vi "pm Main.vi"() -> ()   [LabVIEW 2022 SP3]
doc: "This Continuous Measurement sample project is based on the Queued Message Handler template.\n\nThe Event Handling Loop generates messages based on user interface actions.\n\nThe Message Handling Loop processes messages generated by the Event Handling Loop, or by other messages. There are also Acquisition and Logging message handling loop subVIs, and a chart updating loop."
uses:
  Settings/Settings.ctl
  Acquisition/Hardware Configuration.ctl
  Acquisition/Signal Type.ctl
  Logging/Logging Configuration.ctl
  controls/pm UI Data.ctl
  controls/pm UI State.ctl
  support/Message Queue/Enqueue Message (Single).vi
  support/Message Queue/Enqueue Message (Array).vi
  <vilib>/Utility/error.llb/Error Cluster From Error Code.vi
  <vilib>/ErrorRing/Error Ring.xnode
  Acquisition/pm Acquisition.lvlib
  Logging/pm Logging.lvlib
  Settings/pm Settings.lvlib
  support/User Event - Stop/pm User Event - Stop.lvlib
  support/Message Queue/pm Message Queue.lvlib
  Settings/Settings Dialog.vi
panel:
  out "Message Data":variant
  out "averagedPower":string
  out "instantPower":string
  in  "wavelength":string="976" caption="wavelenght"
  in  "Save":bool
  in  "Start":bool
  in  "Stop":bool
  in  "Settings":bool
  in  "Exit":bool
  out "Status":string
  out "DIstributionP":dbl[][](graph) caption="Intensity Graph"
  out "Data":waveform(dbl)[](graph)
  # "Longueur d'onde"
  # "Yes\nNo\nToaster"
  # "nm"
  # "logo..."
  # "Puissance instantannée"
  # "W"
  # "Puissance moyenne"
  # "W"
  # "Distribution de puissance"
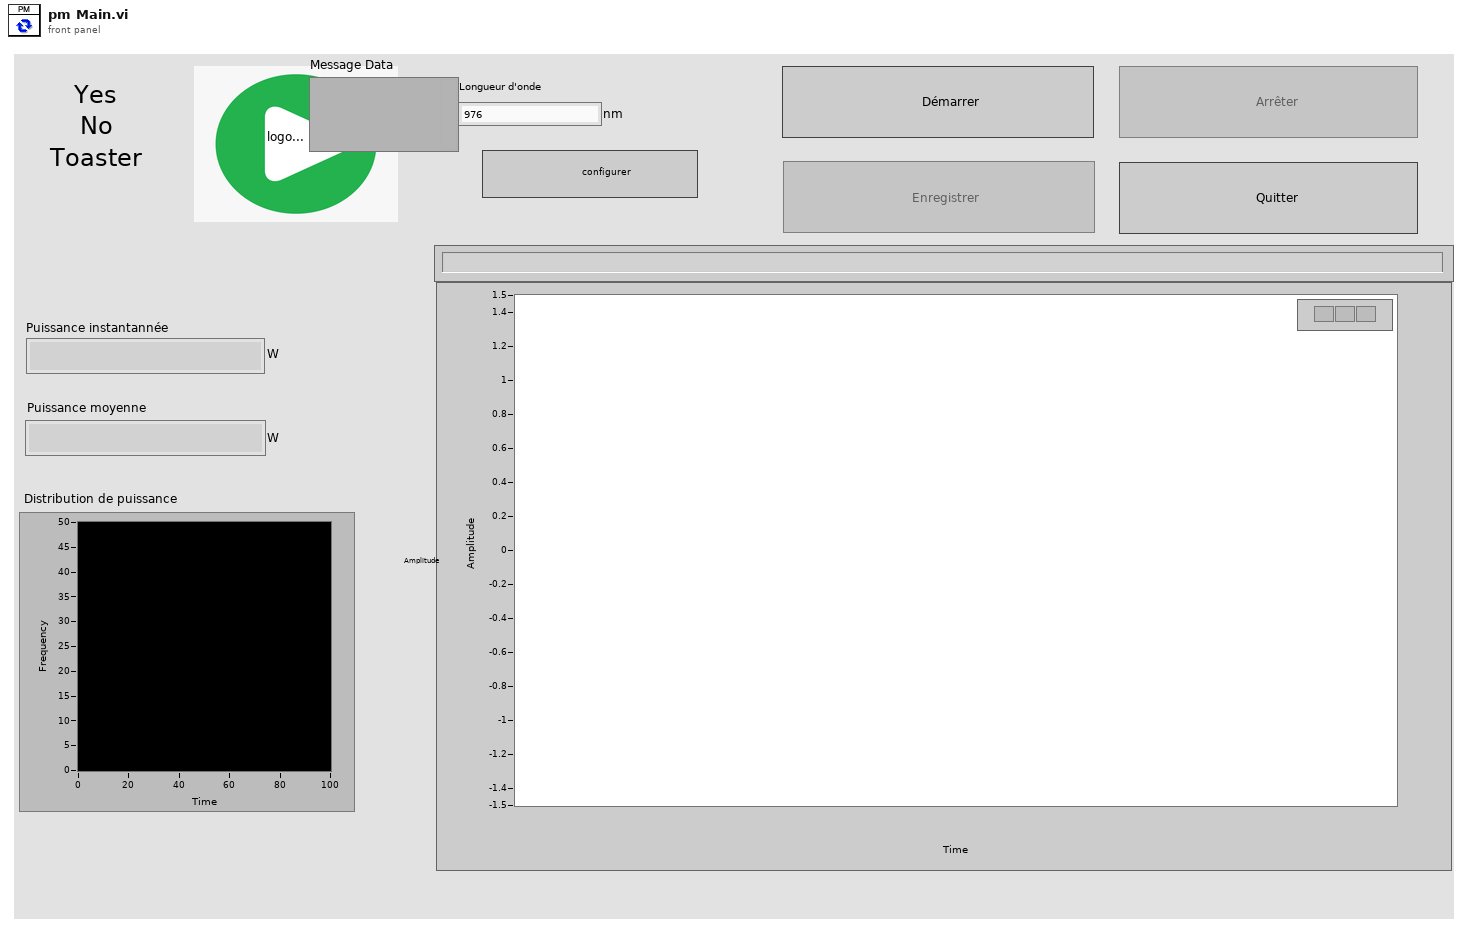
[diagram p1: front panel]
types:
  T1 = typedef "pm UI State.ctl" = enum16{"Idle", "Acquiring and Logging", "Waiting for Exit", "Waiting for Exit (Acq Stopped)", "Waiting for Exit (Log Stopped)", "Waiting for Stop", "Waiting for Stop (Acq Stopped)", "Waiting for Stop (Log Stopped)", "Saving data"}
  T2 = typedef "pm UI Data.ctl" = cluster{"Start Ref":refnum<vi>, "Stop Ref":refnum<vi>, "Settings Ref":refnum<vi>, "Exit Ref":refnum<vi>, "Status Ref":refnum<vi>, "Data Ref":refnum<vi>, "Save":refnum<vi>, "wavelength":refnum<vi>}
  T3 = typedef "pm Settings.lvlib/Settings.ctl" = cluster{"Hardware Configuration":T4, "Logging Configuration":T6}
  T4 = typedef "pm Acquisition.lvlib/Hardware Configuration.ctl" = cluster{"HW Refnum <Replace Me>":string, "Signal Type <Replace Me>":T5}
  T5 = typedef "pm Acquisition.lvlib/Signal Type.ctl" = enum16{"Sine Wave", "Square with Noise"}
  T6 = typedef "pm Logging.lvlib/Logging Configuration.ctl" = cluster{"Log File Base Path":path, "TDMS File Reference":refnum<k34>}
  T7 = typedef "pm Message Queue.lvlib/All Message Queues.ctl" = cluster{"UI":refnum<queue>, "Acquisition":refnum<queue>, "Logging":refnum<queue>}
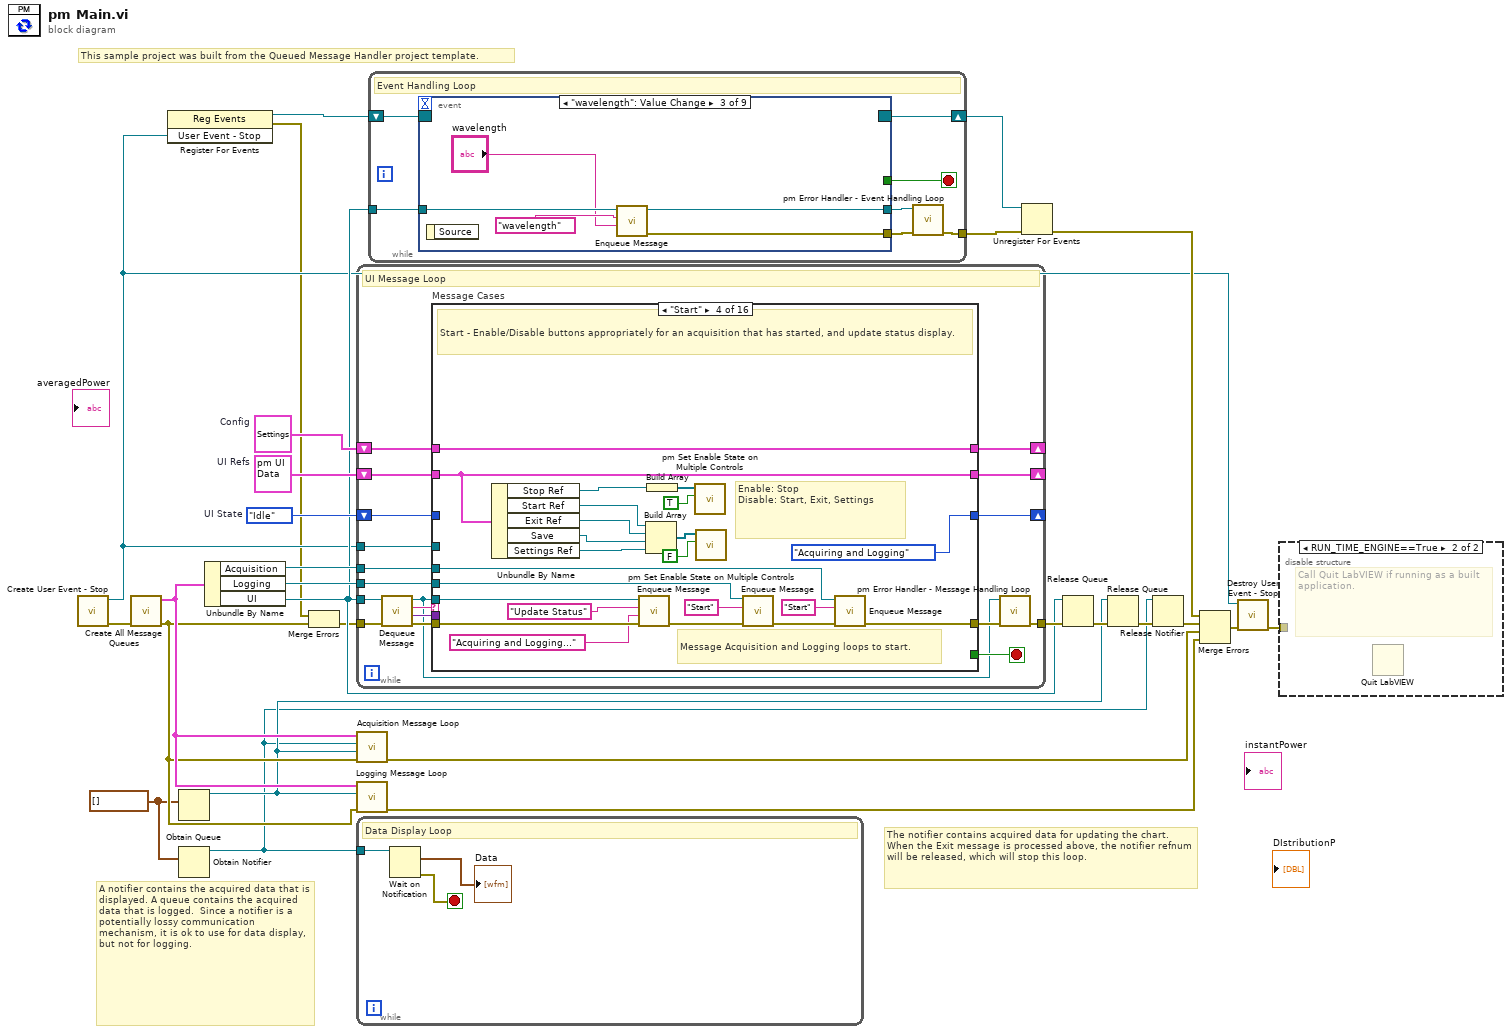
[diagram p0: block diagram]
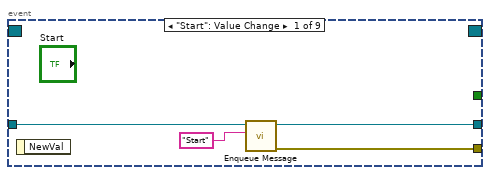
[diagram p3: hidden frame]
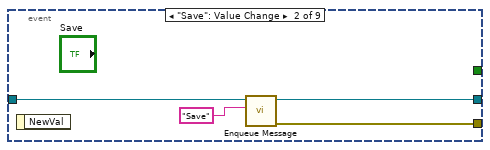
[diagram p4: hidden frame]
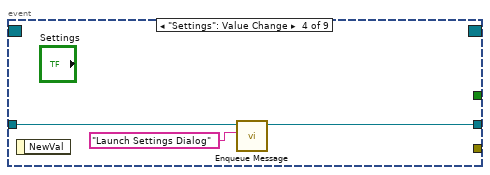
[diagram p5: hidden frame]
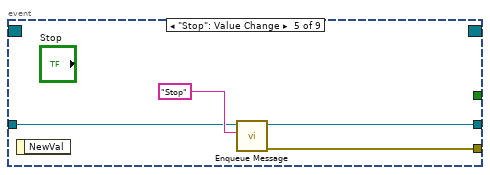
[diagram p6: hidden frame]
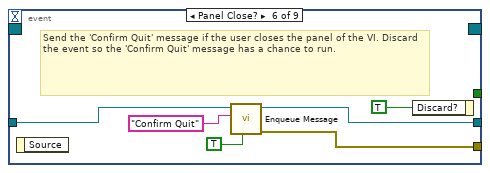
[diagram p7: hidden frame]
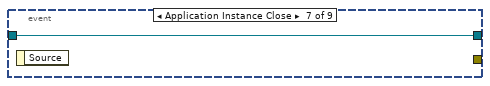
[diagram p8: hidden frame]
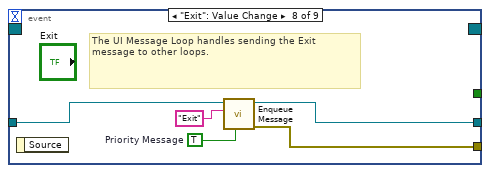
[diagram p9: hidden frame]
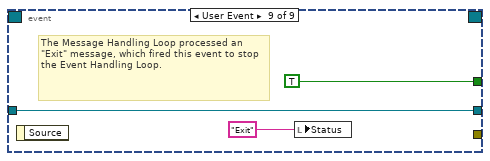
[diagram p10: hidden frame]
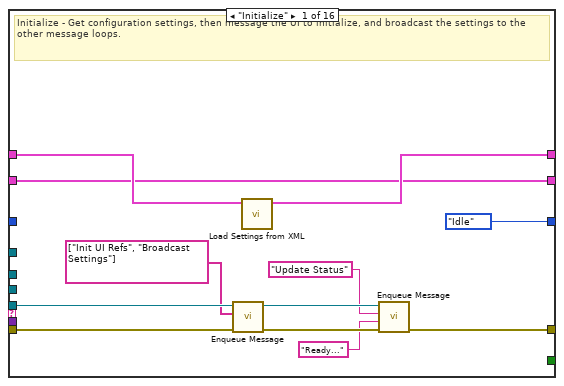
[diagram p11: hidden frame]
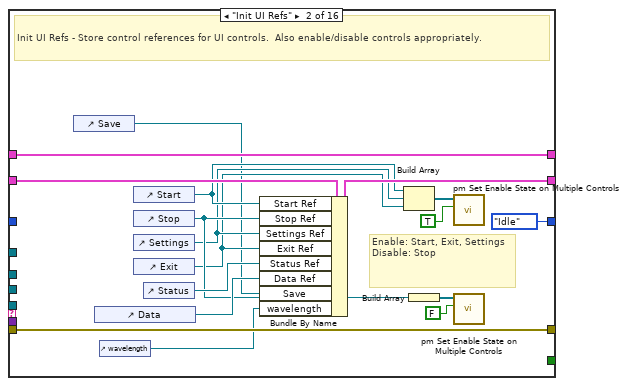
[diagram p12: hidden frame]
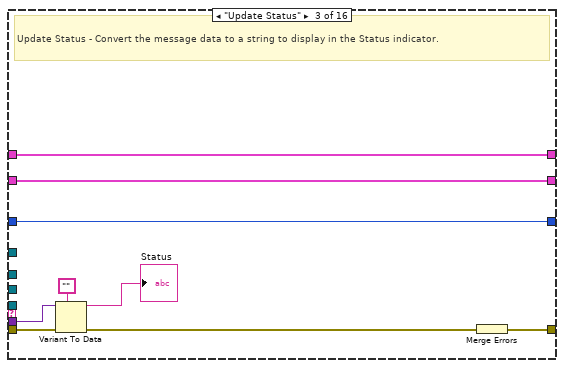
[diagram p13: hidden frame]
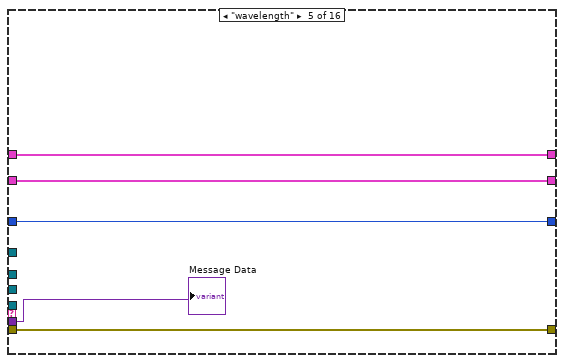
[diagram p14: hidden frame]
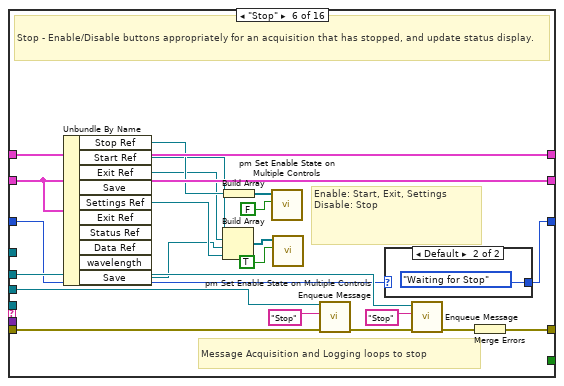
[diagram p15: hidden frame]
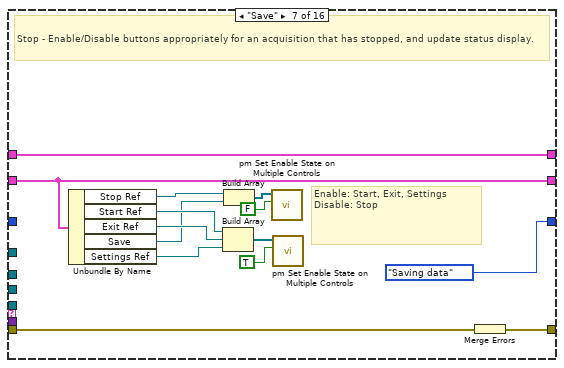
[diagram p17: hidden frame]
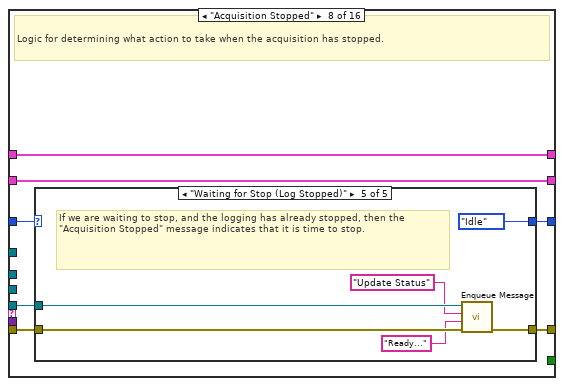
[diagram p18: hidden frame]
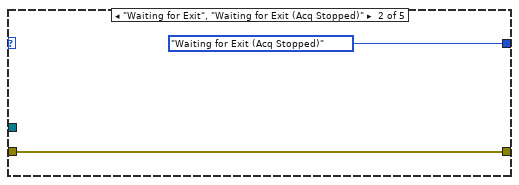
[diagram p20: hidden frame]
diagram:
  w14 = pm_UI_State."Idle"  # UI State
  w5 = waveform(dbl)[] []
  w17 = T2 {"Start Ref"=refnum, "Stop Ref"=refnum, "Settings Ref"=refnum, "Exit Ref"=refnum, "Status Ref"=refnum, "Data Ref"=refnum, "Save"=refnum, "wavelength"=refnum}  # UI Refs
  w20 = T3 {"Hardware Configuration"={"HW Refnum <Replace Me>"="", "Signal Type <Replace Me>"=enum."Sine Wave"}, "Logging Configuration"={"Log File Base Path"=path "", "TDMS File Reference"=refnum}}  # Config
  # "This sample project was built from the Queued Message Handler project template."
  # "A notifier contains the acquired data that is displayed. A queue contains the acquired data that is logged.  Since a notifier is a potentially lossy communication mechanism, it is ok to use for data display, but not for logging."
  # "The notifier contains acquired data for updating the chart. When the Exit message is processed above, the notifier refnum will be released, which will stop this loop."
  n1 = call "Create User Event - Stop.vi"() -> ("error out"=w24:errorcluster, "User Event - Stop"=w3:refnum<user-event>)  [unwired: 10 in]
  n2 = call "Create All Message Queues.vi"("error in (no error)"=w24) -> ("error out"=w21:errorcluster, "Message Queues out"=w23:T7)  [unwired: 9 in]
  n3 = register-events(w3) -> (reference out=w4:refnum<event-registration>, error out=w1:errorcluster)  [unwired: 2 in]
  n4 = Obtain Queue(element data type=w5) -> (queue out=w7:refnum<queue>)  [unwired: 4 in, 2 out]
  n5 = Obtain Notifier(notification data type=w5) -> (notifier out=w6:refnum<notifier>)  [unwired: 3 in, 2 out]
  n6 = Unbundle By Name(w23) -> ("Acquisition"=w16:refnum<queue>, "Logging"=w15:refnum<queue>, "UI"=w12:refnum<queue>)
  n7 = Merge Errors(w1, w21) -> (w2:errorcluster)
  n8 = while {
    tunnel: w12 -> [w39]
    tunnel: w3 -> [w44]
    shift-right: [w38] -> _
    shift-left: w20 -> [w37]
    shift-right: [w35] -> _
    shift-left: w17 -> [w36]
    tunnel: w16 -> [w34]
    tunnel: w15 -> [w33]
    shift-right: [w28] -> _
    shift-left: w14 -> [w29]
    tunnel: w2 -> [w43]
    tunnel: [w32] -> w27
    stop <- w45 stop-if-true
    # "UI Message Loop"
    n9 = call "Dequeue Message.vi"("error in (no error)"=w43, "Message Queue"=w39) -> ("error out"=w42:errorcluster, "Message Data"=w40:variant, "Message"=w41:string, "dup Message Queue"=w30:refnum<queue>)  [unwired: 6 in]
    n10 = case "Message Cases" shown="\"Start\"" w41 {
      selector: w41 -> [_ _ _ _ _ _ _ _ _ _ _ _ _ _ _ w284]
      tunnel: w30 -> [w49 _ _ w106 _ _ _ w151 w176 _ w216 _ w237 _ _ _]
      tunnel: w42 -> [w48 w74 w82 w105 w111 w131 w135 w152 w177 w204 w218 w225 w236 w265 w282 _]
      tunnel: [w53 w74 w83 w88 w111 w132 w148 w149 w174 w210 w211 w228 w235 w275 w281 w283] -> w31
      tunnel: [_ _ _ _ _ _ _ _ _ _ _ _ _ TRUE _ _] -> w45
      tunnel: w40 -> [_ _ w81 _ w107 _ _ _ _ _ _ w229 _ w263 _ _]
      tunnel: w44 -> [_ _ _ _ _ _ _ _ _ _ _ _ _ w276 _ _]
      tunnel: [w56 w73 w77 w104 w110 w130 w147 w155 w180 w208 w215 w233 w240 w274 w280 w287] -> w38
      tunnel: w37 -> [w57 w73 w77 w104 w110 w130 w147 w155 w180 w208 w219 w233 w240 w274 w280 w287]
      tunnel: w36 -> [w50 w72 w76 w101 w108 w129 w146 w154 w179 w202 w213 w232 w239 w273 w279 w286]
      tunnel: [w50 w69 w76 w101 w108 w129 w146 w154 w179 w202 w213 w232 w239 w273 w279 w286] -> w35
      tunnel: w34 -> [_ _ _ w87 _ w116 _ _ _ w201 _ _ _ w272 _ _]
      tunnel: w33 -> [_ _ _ w90 _ w119 _ _ _ w200 _ _ _ w271 _ _]
      tunnel: w29 -> [_ _ w75 _ w109 w113 _ w153 w178 w199 w212 w227 w238 _ w278 w285]
      tunnel: [pm_UI_State."Idle" ("UI State") pm_UI_State."Idle" ("UI State") w75 pm_UI_State."Acquiring and Logging" ("UI State") w109 w114 pm_UI_State."Saving data" ("UI State") w150 w175 w199 w212 w227 w234 pm_UI_State."Idle" ("UI State") w278 w285] -> w28
      frame "Initialize" {
        # "Initialize - Get configuration settings, then message the UI to initialize, and broadcast the settings to the other message loops."
        n11 = call-poly "Enqueue Message.vi"("error in (no error)"=w48, "Message Array"=string[] ["Init UI Refs", "Broadcast Settings"], "Message Queue"=w49) -> ("error out"=w55:errorcluster, "dup Message Queue"=w54:refnum<queue>)  [unwired: 7 in]
        n12 = call "Load Settings from XML.vi"("Settings in"=w57) -> ("Settings out"=w56:T3)  [unwired: 9 in, 1 out]
        n13 = call-poly "Enqueue Message.vi"("error in (no error)"=w55, "Message Data"="Ready..." ("Ready..."), "Message"="Update Status", "Message Queue"=w54) -> ("error out"=w53:errorcluster)  [unwired: 6 in, 1 out]
      }
      frame "Init UI Refs" {
        # "Enable: Start, Exit, Settings\nDisable: Stop"
        # "Init UI Refs - Store control references for UI controls.  Also enable/disable controls appropriately."
        n14 = control-ref of="Save"() -> (w59:refnum<vi>)
        n15 = control-ref of="Data"() -> (w70:refnum<vi>)
        n16 = control-ref of="wavelength"() -> (w58:refnum<vi>)
        n17 = control-ref of="Start"() -> (w63:refnum<vi>)
        n18 = control-ref of="Stop"() -> (w64:refnum<vi>)
        n19 = control-ref of="Settings"() -> (w62:refnum<vi>)
        n20 = control-ref of="Exit"() -> (w61:refnum<vi>)
        n21 = control-ref of="Status"() -> (w71:refnum<vi>)
        n22 = Bundle By Name(cluster=w72, "Start Ref"=w63, "Stop Ref"=w64, "Settings Ref"=w62, "Exit Ref"=w61, "Status Ref"=w71, "Data Ref"=w70, "Save"=w59, "wavelength"=w58) -> (w69:T2)
        n23 = Build Array(w63, w62, w61) -> (w67:refnum<vi>[])
        n24 = Build Array(w64) -> (w66:refnum<vi>[])
        n25 = call "pm Set Enable State on Multiple Controls.vi"("Enable?"=TRUE, "Controls"=w67) -> ()  [unwired: 10 in]
        n26 = call "pm Set Enable State on Multiple Controls.vi"("Enable?"=FALSE, "Controls"=w66) -> ()  [unwired: 10 in]
      }
      frame "Update Status" {
        # "Update Status - Convert the message data to a string to display in the Status indicator."
        n27 = Variant To Data(error in=w82, type="", Variant=w81) -> (data=→"Status":string, error out=w79:errorcluster)
        n28 = Merge Errors(w79) -> (w83:errorcluster)
      }
      frame "Start" {
        # "Message Acquisition and Logging loops to start."
        # "Enable: Stop\nDisable: Start, Exit, Settings"
        # "Start - Enable/Disable buttons appropriately for an acquisition that has started, and update status display."
        n29 = Unbundle By Name(w101) -> ("Stop Ref"=w96:refnum<vi>, "Start Ref"=w95:refnum<vi>, "Exit Ref"=w94:refnum<vi>, "Save"=w84:refnum<vi>, "Settings Ref"=w93:refnum<vi>)
        n30 = call-poly "Enqueue Message.vi"("error in (no error)"=w105, "Message Data"="Acquiring and Logging..." ("Acquiring and Logging..."), "Message"="Update Status", "Message Queue"=w106) -> ("error out"=w92:errorcluster)  [unwired: 6 in, 1 out]
        n31 = Build Array(w95, w94, w84, w93) -> (w99:refnum<vi>[])
        n32 = Build Array(w96) -> (w98:refnum<vi>[])
        n33 = call "pm Set Enable State on Multiple Controls.vi"("Enable?"=TRUE, "Controls"=w98) -> ()  [unwired: 10 in]
        n34 = call "pm Set Enable State on Multiple Controls.vi"("Enable?"=FALSE, "Controls"=w99) -> ()  [unwired: 10 in]
        n35 = call-poly "Enqueue Message.vi"("error in (no error)"=w92, "Message"="Start", "Message Queue"=w90) -> ("error out"=w89:errorcluster)  [unwired: 7 in, 1 out]
        n36 = call-poly "Enqueue Message.vi"("error in (no error)"=w89, "Message"="Start", "Message Queue"=w87) -> ("error out"=w88:errorcluster)  [unwired: 7 in, 1 out]
      }
      frame "wavelength" {
        "Message Data" <- w107
      }
      frame "Stop" {
        # "Message Acquisition and Logging loops to stop"
        # "Enable: Start, Exit, Settings\nDisable: Stop"
        # "Stop - Enable/Disable buttons appropriately for an acquisition that has stopped, and update status display."
        n37 = Unbundle By Name(w129) -> ("Stop Ref"=w124:refnum<vi>, "Start Ref"=w123:refnum<vi>, "Exit Ref"=w122:refnum<vi>, "Settings Ref"=w121:refnum<vi>, "Save"=w112:refnum<vi>)  [unwired: 5 out]
        n38 = Build Array(w123, w122, w112, w121) -> (w127:refnum<vi>[])
        n39 = Build Array(w124) -> (w126:refnum<vi>[])
        n40 = call "pm Set Enable State on Multiple Controls.vi"("Enable?"=FALSE, "Controls"=w126) -> ()  [unwired: 10 in]
        n41 = call "pm Set Enable State on Multiple Controls.vi"("Enable?"=TRUE, "Controls"=w127) -> ()  [unwired: 10 in]
        n42 = call-poly "Enqueue Message.vi"("error in (no error)"=w131, "Message"="Stop", "Message Queue"=w119) -> ("error out"=w118:errorcluster)  [unwired: 7 in, 1 out]
        n43 = case shown="Default" w113 {
          selector: w113 -> [w133 _]
          tunnel: [w133 pm_UI_State."Waiting for Stop" ("UI State")] -> w114
          frame "Waiting for Exit" {
          }
          frame Default {
          }
        }
        n44 = call-poly "Enqueue Message.vi"("error in (no error)"=w118, "Message"="Stop", "Message Queue"=w116) -> ("error out"=w117:errorcluster)  [unwired: 7 in, 1 out]
        n45 = Merge Errors(w117) -> (w132:errorcluster)
      }
      frame "Save" {
        # "Enable: Start, Exit, Settings\nDisable: Stop"
        # "Stop - Enable/Disable buttons appropriately for an acquisition that has stopped, and update status display."
        n46 = Unbundle By Name(w146) -> ("Stop Ref"=w141:refnum<vi>, "Start Ref"=w140:refnum<vi>, "Exit Ref"=w139:refnum<vi>, "Save"=w136:refnum<vi>, "Settings Ref"=w138:refnum<vi>)
        n47 = Build Array(w140, w139, w138) -> (w144:refnum<vi>[])
        n48 = Build Array(w141, w136) -> (w143:refnum<vi>[])
        n49 = call "pm Set Enable State on Multiple Controls.vi"("Enable?"=FALSE, "Controls"=w143) -> ()  [unwired: 10 in]
        n50 = call "pm Set Enable State on Multiple Controls.vi"("Enable?"=TRUE, "Controls"=w144) -> ()  [unwired: 10 in]
        n51 = Merge Errors(w135) -> (w148:errorcluster)
      }
      frame "Acquisition Stopped" {
        # "Logic for determining what action to take when the acquisition has stopped."
        n52 = case shown="\"Waiting for Stop (Log Stopped)\"" w153 {
          selector: w153 -> [w157 _ _ _ _]
          tunnel: w152 -> [w156 w159 w161 w167 w173]
          tunnel: w151 -> [_ _ _ w165 w170]
          tunnel: [w157 pm_UI_State."Waiting for Exit (Acq Stopped)" ("UI State") pm_UI_State."Waiting for Stop (Acq Stopped)" ("UI State") pm_UI_State."Idle" ("UI State") pm_UI_State."Idle" ("UI State")] -> w150
          tunnel: [w156 w159 w161 w166 w171] -> w149
          frame Default {
          }
          frame "Waiting for Exit", "Waiting for Exit (Acq Stopped)" {
          }
          frame "Waiting for Stop", "Waiting for Stop (Acq Stopped)" {
          }
          frame "Waiting for Exit (Log Stopped)" {
            # "If we are waiting to exit, and the logging has already stopped, then the \"Acquisition Stopped\" message indicates that it is time to exit."
            n53 = call-poly "Enqueue Message.vi"("Priority Message? (F)"=TRUE, "error in (no error)"=w167, "Message"="Exit", "Message Queue"=w165) -> ("error out"=w166:errorcluster)  [unwired: 6 in, 1 out]
          }
          frame "Waiting for Stop (Log Stopped)" {
            # "If we are waiting to stop, and the logging has already stopped, then the \"Acquisition Stopped\" message indicates that it is time to stop."
            n54 = call-poly "Enqueue Message.vi"("error in (no error)"=w173, "Message Data"="Ready..." ("Ready..."), "Message"="Update Status", "Message Queue"=w170) -> ("error out"=w171:errorcluster)  [unwired: 6 in, 1 out]
          }
        }
      }
      frame "Logging Stopped" {
        # "Logic for determining what action to take when the logging has stopped."
        n55 = case shown="\"Waiting for Stop\", \"Waiting for Stop (Log Stopped)\"" w178 {
          selector: w178 -> [w182 _ _ _ _]
          tunnel: w177 -> [w181 w184 w186 w192 w195]
          tunnel: w176 -> [_ _ _ w190 w194]
          tunnel: [w182 pm_UI_State."Waiting for Exit (Log Stopped)" ("UI State") pm_UI_State."Waiting for Stop (Log Stopped)" ("UI State") pm_UI_State."Idle" ("UI State") pm_UI_State."Idle" ("UI State")] -> w175
          tunnel: [w181 w184 w186 w191 w193] -> w174
          frame Default {
          }
          frame "Waiting for Exit", "Waiting for Exit (Log Stopped)" {
          }
          frame "Waiting for Stop", "Waiting for Stop (Log Stopped)" {
          }
          frame "Waiting for Exit (Acq Stopped)" {
            # "If we are waiting to exit, and the acquisition has already stopped, then the \"Logging Stopped\" message indicates that it is time to exit."
            n56 = call-poly "Enqueue Message.vi"("Priority Message? (F)"=TRUE, "error in (no error)"=w192, "Message"="Exit", "Message Queue"=w190) -> ("error out"=w191:errorcluster)  [unwired: 6 in, 1 out]
          }
          frame "Waiting for Stop (Acq Stopped)" {
            # "If we are waiting to stop, and the acquisition has already stopped, then the \"Logging Stopped\" message indicates that it is time to stop."
            n57 = call-poly "Enqueue Message.vi"("error in (no error)"=w195, "Message Data"="Ready..." ("Ready..."), "Message"="Update Status", "Message Queue"=w194) -> ("error out"=w193:errorcluster)  [unwired: 6 in, 1 out]
          }
        }
      }
      frame "Broadcast settings" {
        w203 = "Update Settings" ("Message")
        # "Broadcast settings - Send the 'Update Settings' message to the Logging and Acquisition message loops."
        n58 = Unbundle By Name(w208) -> ("Hardware Configuration"=w207:T4, "Logging Configuration"=w206:T6)
        n59 = call-poly "Enqueue Message.vi"("Message Data"=w207, "Message"=w203, "Message Queue"=w201) -> ("error out"=w209:errorcluster)  [unwired: 7 in, 1 out]
        n60 = call-poly "Enqueue Message.vi"("error in (no error)"=w209, "Message Data"=w206, "Message"=w203, "Message Queue"=w200) -> ("error out"=w205:errorcluster)  [unwired: 6 in, 1 out]
        n61 = Merge Errors(w205, w204) -> (w210:errorcluster)
      }
      frame "Launch Settings Dialog" {
        # "Launch Settings Dialog - Launch the Settings Dialog when the user clicks the 'Settings' button."
        n62 = call-by-ref "?"("error in (no error)"=w218, "Settings in"=w219) -> ("error out"=w214:errorcluster, "Cancelled?"=w217:bool, "Settings out"=w215:T3)  [unwired: 8 in, 3 out]
        n63 = case shown="False" w217 {
          tunnel: w216 -> [w223 _]
          tunnel: w214 -> [w222 w224]
          tunnel: [w221 w224] -> w211
          frame False {
            n64 = call-poly "Enqueue Message.vi"("error in (no error)"=w222, "Message"="Broadcast Settings", "Message Queue"=w223) -> ("error out"=w221:errorcluster)  [unwired: 7 in, 1 out]
          }
          frame True {
          }
        }
      }
      frame "Error" {
        # "Error - Display an error dialog. This message is sent by the \"Error Handler\" VIs at the end of other loops in this application."
        n65 = Variant To Data(error in=w225, type=errorcluster {"status"=FALSE, "code"=0, "source"=""} ("error constant"), Variant=w229) -> (data=w226:errorcluster, error out=w230:errorcluster)
        n66 = call <vilib>:"Simple Error Handler.vi"("error in (no error)"=w226) -> ()  [unwired: 4 in, 5 out]
        n67 = Merge Errors(w230) -> (w228:errorcluster)
      }
      frame "Confirm Quit" {
        # "Confirm Quit - Message that can confirm whether or not the user wants to exit the application."
        n68 = case shown="\"Acquiring and Logging\"" w238 {
          tunnel: w237 -> [w246 w250]
          tunnel: w236 -> [w245 w249]
          tunnel: [w244 w248] -> w235
          tunnel: [pm_UI_State."Idle" ("UI State") w247] -> w234
          frame Default {
            # "If 'Confirm Quit' comes in while the system is idle, there is no need for a confirmation message."
            n69 = call-poly "Enqueue Message.vi"("Priority Message? (F)"=TRUE, "error in (no error)"=w245, "Message"="Exit", "Message Queue"=w246) -> ("error out"=w244:errorcluster)  [unwired: 6 in, 1 out]
          }
          frame "Acquiring and Logging" {
            n70 = Two Button Dialog(message="Are you sure you want to quit while the acquisition is running?" ("Confirm Quit Message"), 1:"No" ("No"), 2:"Yes" ("Yes")) -> (T button?=w251:bool)
            n71 = case shown="True" w251 {
              tunnel: w250 -> [_ w260]
              tunnel: w249 -> [w256 w261]
              tunnel: [w256 w259] -> w248
              tunnel: [pm_UI_State."Acquiring and Logging" ("UI State") pm_UI_State."Waiting for Exit" ("UI State")] -> w247
              frame False {
                # "User did not want to quit."
              }
              frame True {
                n72 = call-poly "Enqueue Message.vi"("error in (no error)"=w261, "Message"="Stop", "Message Queue"=w260) -> ("error out"=w259:errorcluster)  [unwired: 7 in, 1 out]
              }
            }
          }
        }
      }
      frame "Exit" {
        w267 = TRUE ("Priority Message? (F)")
        w268 = "Exit" ("Message")
        # "Popup an error dialog if 'Exit' was called as a result of an error."
        # "Stop the VI"
        # "Exit - Send Exit messages to the Acquisition and Logging loops, and fire the user event to stop the Event Handling Loop."
        n73 = Variant To Data(type=errorcluster {"status"=FALSE, "code"=0, "source"=""} ("error constant"), Variant=w263) -> (data=w262:errorcluster)  [unwired: 1 in, 1 out]
        n74 = call <vilib>:"Simple Error Handler.vi"("error in (no error)"=w262) -> ()  [unwired: 4 in, 5 out]
        n75 = call-poly "Enqueue Message.vi"("Priority Message? (F)"=w267, "error in (no error)"=w265, "Message"=w268, "Message Queue"=w272) -> ("error out"=w269:errorcluster)  [unwired: 6 in, 1 out]
        n76 = call-poly "Enqueue Message.vi"("Priority Message? (F)"=w267, "error in (no error)"=w269, "Message"=w268, "Message Queue"=w271) -> ("error out"=w266:errorcluster)  [unwired: 6 in, 1 out]
        n77 = call "Fire User Event - Stop.vi"("error in (no error)"=w266, "User Event - Stop"=w276) -> ("error out"=w275:errorcluster)  [unwired: 9 in]
      }
      frame "---Copy This Frame---" {
        # "Duplicate this frame when creating new messages.  Change this comment in the duplicated frame to describe this message."
        n78 = Merge Errors(w282) -> (w281:errorcluster)
      }
      frame Default {
        # "'Default' case only runs if there is a message that isn't defined in any of the other cases.  Output a programming error."
        n79 = xnode "Error Ring"("parameter 0"=w284) -> ("error out"=w283:errorcluster)
      }
    }
    n80 = call "pm Error Handler - Message Handling Loop.vi"("error in (no error)"=w31, "Message Queue"=w30) -> ("dup error in"=w32:errorcluster)  [unwired: 8 in, 1 out]
  }
  n81 = call "Acquisition Message Loop.vi"("error in (no error)"=w21, "Data Queue"=w7, "Data Notifier"=w6, "Message Queues"=w23) -> ("error out"=w25:errorcluster)  [unwired: 7 in]
  n82 = call "Logging Message Loop.vi"("error in (no error)"=w21, "Data Queue"=w7, "Message Queues"=w23) -> ("error out"=w22:errorcluster)  [unwired: 8 in]
  n83 = while "Data Display Loop" {
    tunnel: w6 -> [w297]
    stop <- w295 stop-if-true
    # "Data Display Loop"
    n84 = Wait on Notification(notifier=w297) -> (notification=→"Data":waveform(dbl)[], error out=w295:errorcluster)  [unwired: 3 in, 2 out]
  }
  n85 = while {
    tunnel: w12 -> [w303]
    tunnel: [w300] -> w26
    shift-right: [w302] -> w18
    shift-left: w4 -> [w304]
    stop <- w301 stop-if-true
    # "Event Handling Loop"
    n86 = event shown="[2] \"wavelength\": Value Change" {
      selector: w304 -> [_ _ _ _ _ _ _ _ _]
      dyn-events: [_ _ _ _ _ _ _ _ _] -> w302
      timeout: _ -> [_ _ _ _ _ _ _ _ _]
      tunnel: [_ _ _ _ _ _ _ _ TRUE ("Discard?")] -> w301
      tunnel: w303 -> [w308 w312 w317 w319 w323 w328 w331 w333 w337]
      tunnel: [w306 w310 w315 _ w322 w326 _ w336 _] -> w299
      tunnel: [w305 w309 w316 w318 w321 w327 w331 w332 w337] -> w298
      event "Start": Value Change {
        n87 = event-data() -> ()  [unwired: 1 in, 1 out]
        n88 = call-poly "Enqueue Message.vi"("Message"="Start", "Message Queue"=w308) -> ("error out"=w306:errorcluster, "dup Message Queue"=w305:refnum<queue>)  [unwired: 8 in]
      }
      event "Save": Value Change {
        n89 = event-data() -> ()  [unwired: 1 in, 1 out]
        n90 = call-poly "Enqueue Message.vi"("Message"="Save", "Message Queue"=w312) -> ("error out"=w310:errorcluster, "dup Message Queue"=w309:refnum<queue>)  [unwired: 8 in]
      }
      event "wavelength": Value Change {
        n91 = event-data() -> ()  [unwired: 1 in, 1 out]
        n92 = call-poly "Enqueue Message.vi"("Message Data"="wavelength", "Message"="wavelength", "Message Queue"=w317) -> ("error out"=w315:errorcluster, "dup Message Queue"=w316:refnum<queue>)  [unwired: 7 in]
      }
      event "Settings": Value Change {
        n93 = event-data() -> ()  [unwired: 1 in, 1 out]
        n94 = call-poly "Enqueue Message.vi"("Message"="Launch Settings Dialog", "Message Queue"=w319) -> ("dup Message Queue"=w318:refnum<queue>)  [unwired: 8 in, 1 out]
      }
      event "Stop": Value Change {
        n95 = event-data() -> ()  [unwired: 1 in, 1 out]
        n96 = call-poly "Enqueue Message.vi"("Message"="Stop", "Message Queue"=w323) -> ("error out"=w322:errorcluster, "dup Message Queue"=w321:refnum<queue>)  [unwired: 8 in]
      }
      event Panel Close? {
        # "Send the 'Confirm Quit' message if the user closes the panel of the VI. Discard the event so the 'Confirm Quit' message has a chance to run."
        n97 = event-data() -> ()  [unwired: 1 in, 1 out]
        n98 = call-poly "Enqueue Message.vi"("Priority Message? (F)"=TRUE, "Message"="Confirm Quit", "Message Queue"=w328) -> ("error out"=w326:errorcluster, "dup Message Queue"=w327:refnum<queue>)  [unwired: 7 in]
        n99 = event-data("Discard?"=TRUE) -> ()  [unwired: 1 in, 1 out]
      }
      event Application Instance Close {
        n100 = event-data() -> ()  [unwired: 1 in, 1 out]
      }
      event "Exit": Value Change {
        w334 = TRUE  # Priority Message
        # "The UI Message Loop handles sending the Exit message to other loops."
        n101 = event-data() -> ()  [unwired: 1 in, 1 out]
        n102 = call-poly "Enqueue Message.vi"("Priority Message? (F)"=w334, "Message"="Exit", "Message Queue"=w333) -> ("error out"=w336:errorcluster, "dup Message Queue"=w332:refnum<queue>)  [unwired: 7 in]
      }
      event User Event {
        # "The Message Handling Loop processed an \"Exit\" message, which fired this event to stop the Event Handling Loop."
        n103 = event-data() -> ()  [unwired: 1 in, 1 out]
        n104 = local write "Status"("Exit" ("Exit String")) -> ()
      }
    }
    n105 = call "pm Error Handler - Event Handling Loop.vi"("error in (no error)"=w299, "Message Queue"=w298) -> ("dup error in"=w300:errorcluster)  [unwired: 8 in, 1 out]
  }
  n106 = Unregister For Events(event registration refnum=w18, error in=w26) -> (error out=w19:errorcluster)
  n107 = Release Queue(queue=w12, error in (no error)=w27) -> (error out=w10:errorcluster)  [unwired: 1 in, 2 out]
  n108 = Release Queue(queue=w7, error in (no error)=w10) -> (error out=w9:errorcluster)  [unwired: 1 in, 2 out]
  n109 = Release Notifier(notifier=w6, error in (no error)=w9) -> (error out=w8:errorcluster)  [unwired: 1 in, 2 out]
  n110 = Merge Errors(w19, w8, w25, w22) -> (w13:errorcluster)
  n111 = call "Destroy User Event - Stop.vi"("error in (no error)"=w13, "User Event - Stop"=w3) -> ("error out"=w11:errorcluster)  [unwired: 9 in]
  n112 = disable-structure shown="RUN_TIME_ENGINE==True" {
    disable-tunnel: w11 -> [_ _]
    frame condition #0 (active) {
    }
    frame condition #1 {
      # "Call Quit LabVIEW if running as a built application."
      n113 = Quit LabVIEW() -> ()  [unwired: 1 in]
    }
  }
